vi "CopyOverlay.vi"(7 "Groups":string[](array[string]), 8 "error in":errorcluster, 10 "Dst Reference In":T1, 11 "Src Reference In":T1) -> (0 "error out":errorcluster, 3 "Dst Reference Out":T1)   [LabVIEW 2024, in "OpenLvVision_Overlays.lvlib"]
doc: "Copies an image overlay from a source to a destination image. If the destination image already contains an overlay, this VI combines the source overlay with the pre-existing one."
uses:
  OpenLvVision_Overlays.lvlib
  <vilib>/OpenLvVision/OpenLvVision_Image/Management/TypeDef/OLV Image.ctl
  <vilib>/OpenLvVision/OpenLvVision_Image/Management/OLV Management.lvlib
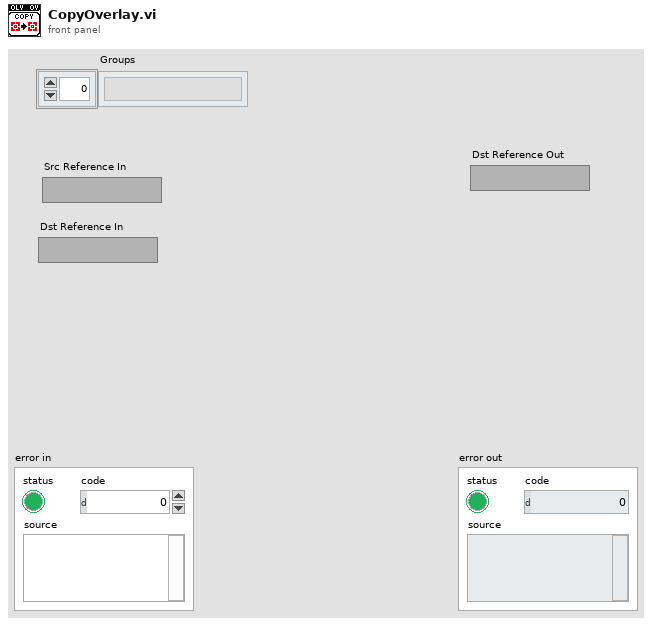
[diagram p1: front panel]
types:
  T1 = typedef "OLV OpenLvVision_Image.lvlib/OLV Management.lvlib/OLV Image.ctl" = refnum<image>
  T2 = typedef "IMAQ Image.ctl" = refnum<image>
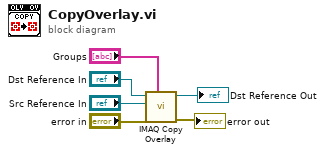
[diagram p0: block diagram]
diagram:
  n1 = call "IMAQ Copy Overlay"("Groups"="Groups", "error in (no error)"="error in", "Image Dst"="Src Reference In", "Image Src"="Dst Reference In") -> ("error out"=→"error out":errorcluster, "Image Dst Out"=→"Dst Reference Out":T2)  [unwired: 6 in]
